vi "Open CHM documentation.vi"(8 "error in":errorcluster) -> (0 "error out":errorcluster)   [LabVIEW 2016]
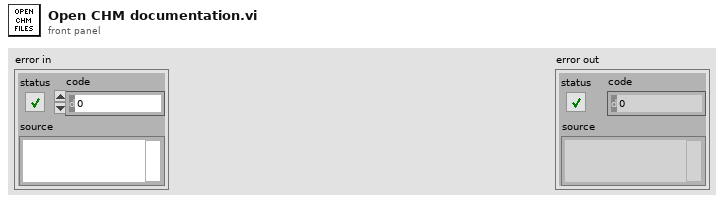
[diagram p1: front panel]
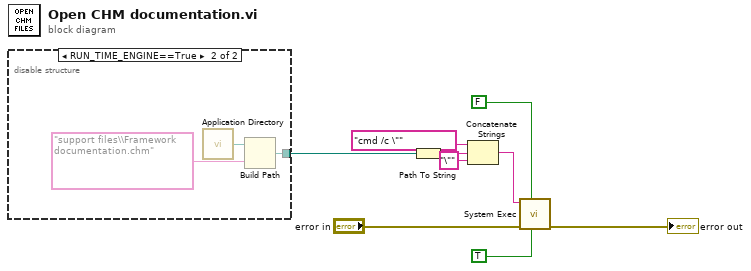
[diagram p0: block diagram]
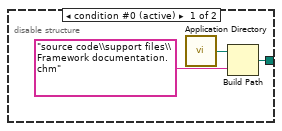
[diagram p2: hidden frame]
diagram:
  n1 = disable-structure shown="RUN_TIME_ENGINE==True" {
    disable-tunnel: [w10 w13] -> w9
    frame condition #0 (active) {
      n2 = call <vilib>:"Application Directory.vi"() -> ("Application Directory"=w11:path)
      n3 = Build Path(base path=w11, name or relative path="source code\\support files\\Framework documentation.chm") -> (appended path=w10:path)
    }
    frame condition #1 {
      n4 = call <vilib>:"Application Directory.vi"() -> ("Application Directory"=w14:path)
      n5 = Build Path(base path=w14, name or relative path="support files\\Framework documentation.chm") -> (appended path=w13:path)
    }
  }
  n6 = Path To String(path=w9) -> (string=w8:string)
  n7 = Concatenate Strings("cmd /c \"", w8, "\"" ("string")) -> (w5:string)
  n8 = call <vilib>:"System Exec.vi"("run minimized? (F)"=TRUE, "wait until completion? (T)"=FALSE, "error in (no error)"="error in", "command line"=w5) -> ("error out"=→"error out":errorcluster)  [unwired: 4 in, 3 out]
